vi "set control size.vi"(8 "error in (no error)":errorcluster, 10 "Size":T1, 11 "String Control in":refnum<class "String Control.lvclass">) -> (0 "error out":errorcluster, 3 "String Control out":refnum<class "String Control.lvclass">)   [LabVIEW 2010, in "String Control.lvclass"]
uses:
  String Control.lvclass
  <vilib>/Utility/miscctls.llb/LVBoundsTypeDef.ctl
  String Control.lvclass/String Control.ctl
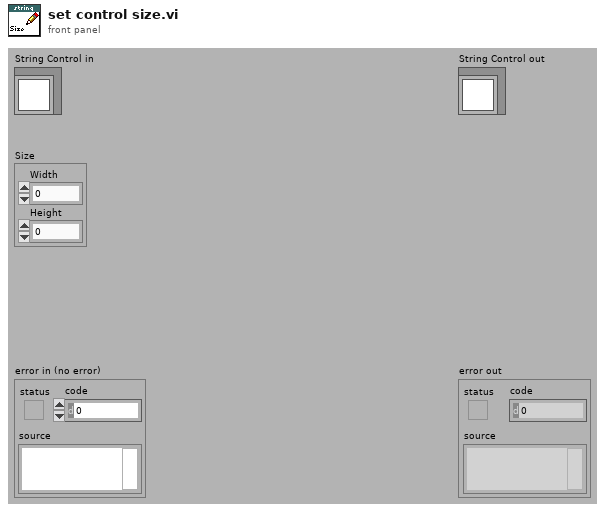
[diagram p1: front panel]
types:
  T1 = typedef "LVBoundsTypeDef.ctl" = cluster{"Width":u32, "Height":u32}
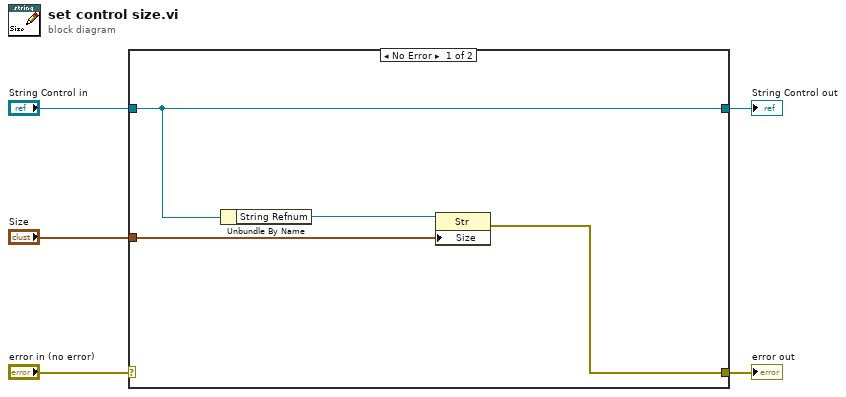
[diagram p0: block diagram]
diagram:
  n1 = case shown="No Error" "error in (no error)" {
    selector: "error in (no error)" -> [_ w11]
    tunnel: [w8 w11] -> w4
    tunnel: [w7 w10] -> w2
    tunnel: "String Control in" -> [w7 w10]
    tunnel: "Size" -> [w9 _]
    frame No Error {
      n2 = Unbundle By Name(w7) -> ("String Refnum"=w6:refnum<vi>)
      n3 = property class="Str"(reference=w6, "Size"=w9) -> (error out=w8:errorcluster)  [unwired: 1 in, 1 out]
    }
    frame Error {
    }
  }
  "error out" <- w4
  "String Control out" <- w2
